vi "GetDistance.vi"(10 "sensors list":string[](array[string]), 11 "packet in":u8[](array[numeric])) -> (3 "distance (mm)":dbl)   [LabVIEW 2018]
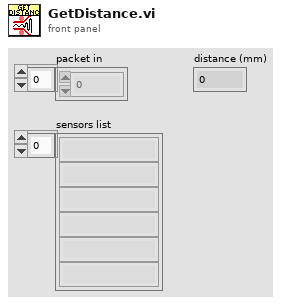
[diagram p1: front panel]
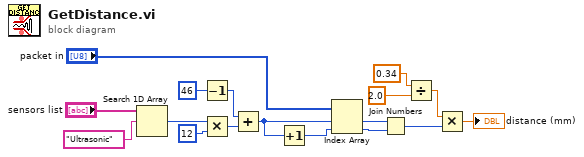
[diagram p0: block diagram]
diagram:
  n1 = Search 1D Array(1D array="sensors list", element="Ultrasonic") -> (index of element=w6:i32)  [unwired: 1 in]
  n2 = Decrement(x=46) -> (x-1=w8:i32)
  n3 = Multiply(x=w6, y=12) -> (x*y=w7:i32)
  n4 = Add(x=w8, y=w7) -> (x+y=w9:i32)
  n5 = Increment(x=w9) -> (x+1=w10:i32)
  n6 = Index Array(array="packet in", index #1=w9, index #2=w10) -> (element #1=w12:u8, element #2=w11:u8)
  n7 = Join Numbers(hi=w12, lo=w11) -> ((hi.lo)=w15:u16)
  n8 = Divide(x=0.34, y=2.0 ("x")) -> (x/y=w16:dbl)
  n9 = Multiply(x=w16, y=w15) -> (x*y=→"distance (mm)":dbl)
